vi "Deadband.vi"(2 "Deadband":dbl, 3 "Input":dbl) -> (0 "In Deadband":bool, 1 "Output":dbl)   [LabVIEW 2012]
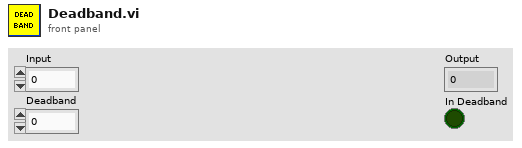
[diagram p1: front panel]
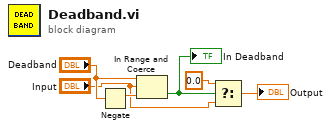
[diagram p0: block diagram]
diagram:
  n1 = Negate(x="Deadband") -> (-x=w6:dbl)
  n2 = In Range and Coerce(upper limit="Deadband", x="Input", lower limit=w6) -> (In Range?=w1:bool)  [unwired: 1 out]
  "In Deadband" <- w1
  n3 = Select(t=0.0, s=w1, f="Input") -> (s? t:f=→"Output":dbl)
